vi "Vertical Rectangle Comparison.vi"(6 "Line Border":cluster{"Top":dbl, "Bottom":dbl}={"Top"=6.0, "Bottom"=1.0}, 9 "Second":dbl[](array[numeric]), 11 "First":dbl[](array[numeric])) -> (0 "Rect":T1, 1 "Line":T1, 3 "Scores":T2)   [LabVIEW 2016]
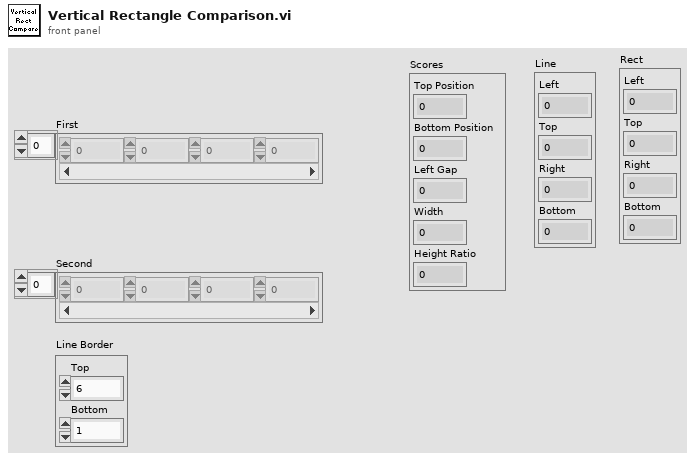
[diagram p1: front panel]
types:
  T1 = cluster{"Left":dbl, "Top":dbl, "Right":dbl, "Bottom":dbl}
  T2 = cluster{"Top Position":dbl, "Bottom Position":dbl, "Left Gap":dbl, "Width":dbl, "Height Ratio":dbl}
  T3 = cluster{"[0]":dbl, "[1]":dbl, "[2]":dbl, "[3]":dbl}
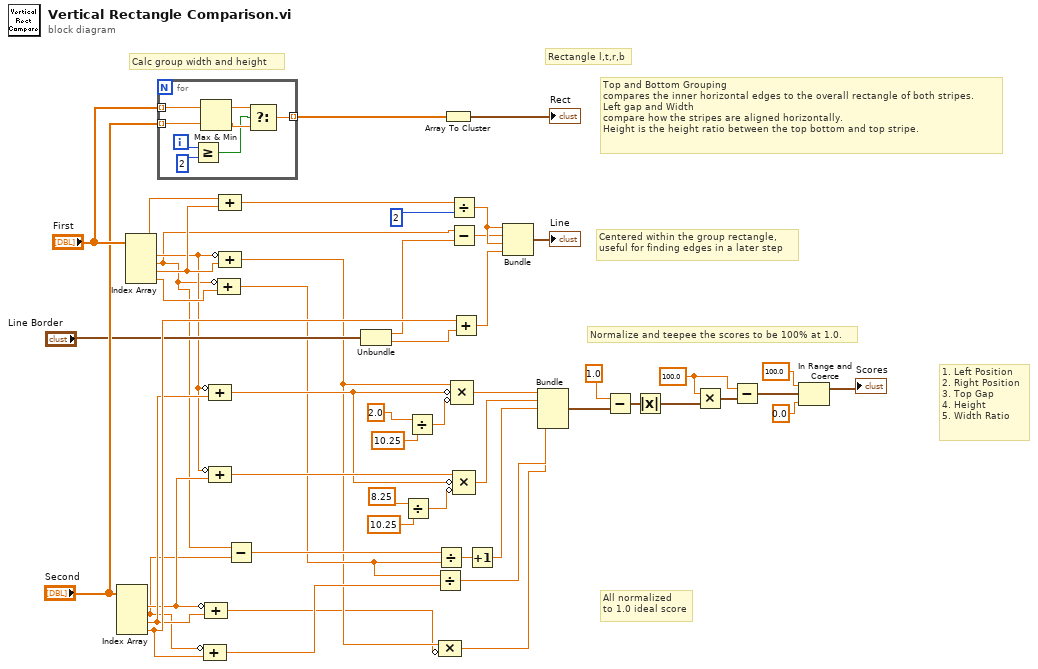
[diagram p0: block diagram]
diagram:
  w30 = 100.0 ("x/y")
  # "1. Left Position\n2. Right Position\n3. Top Gap\n4. Height\n5. Width Ratio"
  # "Centered within the group rectangle,\nuseful for finding edges in a later step"
  # "All normalized\nto 1.0 ideal score"
  # "Normalize and teepee the scores to be 100% at 1.0."
  # "Top and Bottom Grouping\ncompares the inner horizontal edges to the overall rectangle of both stripes.\nLeft gap and Width\ncompare how the stripes are aligned horizontally.\nHeight is the height ratio between the top bottom and top stripe."
  # "Calc group width and height"
  # "Rectangle l,t,r,b"
  n1 = Index Array(array="Second") -> (element #1=w12:dbl, element #2=w8:dbl, element #3=w15:dbl, element #4=w22:dbl)  [unwired: 4 in]
  n2 = Index Array(array="First") -> (element #1=w11:dbl, element #2=w9:dbl, element #3=w44:dbl, element #4=w45:dbl)  [unwired: 4 in]
  n3 = for {
    tunnel: "First" -> [w58] mode=indexing
    tunnel: "Second" -> [w57] mode=indexing
    tunnel: [w51] -> w36 mode=indexing
    i -> [w55]
    n4 = Greater Or Equal?(x=w55, y=2) -> (x >= y?=w52:bool)
    n5 = Max & Min(x=w58, y=w57) -> (max(x,y)=w54:dbl, min(x,y)=w53:dbl)
    n6 = Select(t=w54, s=w52, f=w53) -> (s? t:f=w51:dbl)
  }
  n7 = Compound Arithmetic op=ADD(invert w8, w22) -> (w6:dbl)
  n8 = Compound Arithmetic op=ADD(invert w12, w15) -> (w4:dbl)
  n9 = Compound Arithmetic op=ADD(invert w11, w15) -> (w20:dbl)
  n10 = Compound Arithmetic op=ADD(invert w11, w12) -> (w21:dbl)
  n11 = Compound Arithmetic op=ADD(invert w9, w45) -> (w7:dbl)
  n12 = Compound Arithmetic op=ADD(w11, w44) -> (w43:dbl)
  n13 = Compound Arithmetic op=ADD(invert w11, w44) -> (w5:dbl)
  n14 = Subtract(x=w9, y=w8) -> (x-y=w50:dbl)
  n15 = Unbundle("Line Border") -> ("Top"=w16:dbl, "Bottom"=w17:dbl)
  n16 = Divide(x=8.25, y=10.25) -> (x/y=w1:dbl)
  n17 = Divide(x=2.0, y=10.25) -> (x/y=w10:dbl)
  n18 = Divide(x=w7, y=w6) -> (x/y=w48:dbl)
  n19 = Divide(x=w50, y=w7) -> (x/y=w46:dbl)
  n20 = Compound Arithmetic op=MULTIPLY(w5, invert w4) -> (w47:dbl)
  n21 = Array To Cluster(array=w36) -> (cluster=→"Rect":T3)
  n22 = Divide(x=w43, y=2) -> (x/y=w42:dbl)
  n23 = Subtract(x=w9, y=w16) -> (x-y=w40:dbl)
  n24 = Add(x=w22, y=w17) -> (x+y=w34:dbl)
  n25 = Compound Arithmetic op=MULTIPLY(w5, invert w20, invert w10) -> (w49:dbl)
  n26 = Compound Arithmetic op=MULTIPLY(w21, invert w20, invert w1) -> (w19:dbl)
  n27 = Increment(x=w46) -> (x+1=w33:dbl)
  n28 = Bundle(w42, w40, w42, w34) -> (→"Line":cluster{dbl, dbl, dbl, dbl})  [unwired: 1 in]
  n29 = Bundle(w49, w19, w33, w48, w47) -> (w24:cluster{dbl, dbl, dbl, dbl, dbl})  [unwired: 1 in]
  n30 = Subtract(x=1.0 ("y"), y=w24) -> (x-y=w28:cluster{dbl, dbl, dbl, dbl, dbl})
  n31 = Absolute Value(x=w28) -> (abs(x)=w31:cluster{dbl, dbl, dbl, dbl, dbl})
  n32 = Multiply(x=w30, y=w31) -> (x*y=w32:cluster{dbl, dbl, dbl, dbl, dbl})
  n33 = Subtract(x=w30, y=w32) -> (x-y=w27:cluster{dbl, dbl, dbl, dbl, dbl})
  n34 = In Range and Coerce(upper limit=100.0, x=w27, lower limit=0.0) -> (coerced(x)=→"Scores":cluster{dbl, dbl, dbl, dbl, dbl})  [unwired: 1 out]
